vi "Read state.vi"(11 "IModel in":refnum<class "IModel.lvclass">) -> (2 "DetailedState":T1, 3 "IModel out":refnum<class "IModel.lvclass">)   [LabVIEW 2016, in "IModel.lvclass"]
uses:
  IModel.lvclass
  ts_sallv_sedspectrometer/DataTypes/logevent_detailedState.ctl
  ts_sallv_sedspectrometer/SALLV_sedSpectrometer.lvlib
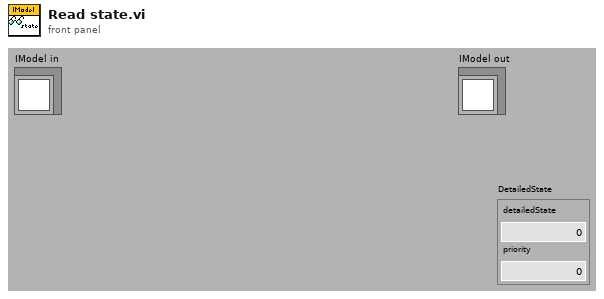
[diagram p1: front panel]
types:
  T1 = typedef "SALLV_sedSpectrometer.lvlib/logevent_detailedState.ctl" = cluster{"detailedState":i32, "priority":i32}
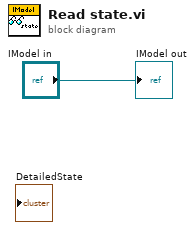
[diagram p0: block diagram]
diagram:
  "IModel out" <- "IModel in"
